vi "Periodic Tasks.vi"() -> ()   [LabVIEW 2012]
doc: "This VI runs in parallel to other tasks. It can contain as many user-defined periodic loops as you need. These can carry out PID or other sorts of timed response."
uses:
  <vilib>/Rock Robotics/WPI/Joystick/WPI_JoystickButtonState.ctl
  <vilib>/Rock Robotics/SystemInterfaces/Utilities/FPGA_UtilitiesLED Source.ctl
  <vilib>/Rock Robotics/SystemInterfaces/Utilities/FPGA_UtilitiesLED State.ctl
  <vilib>/Rock Robotics/WPI/Compressor/WPI_CompressorGetSetRefNum.vi
  Robot Global Data.vi
  <vilib>/Rock Robotics/WPI/RobotDrive/WPI_RobotDriveArcadeDrive_Standard(NoSaturation).vi
  <vilib>/Rock Robotics/WPI/Joystick/WPI_JoystickGetSetRefNum.vi
  <vilib>/Rock Robotics/WPI/RobotDrive/WPI_RobotDriveGetSetRefNum.vi
  <vilib>/Rock Robotics/WPI/Solenoid/WPI_SolenoidSetEnum.vi
  <vilib>/Rock Robotics/WPI/Solenoid/WPI_SolenoidValue.ctl
  <vilib>/Rock Robotics/Network Tables/SD Read Boolean.vi
panel:
  out "y":dbl
  out "x":dbl
  out "Axes":T1
  out "Climber operation":u64
  out "s2b":dbl
  out "s2a":dbl
  out "s1b":dbl
  out "s1a":dbl
  out "Buttons 2":T2
  out "Climber Arm Position":dbl
  out "Right Rate":dbl
  out "Left Rate":dbl
  out "Next Value":dbl
  out "Output 2":dbl
  out "Output":dbl
  out "axis 2 (y)":dbl
  out "Drive Ramp Constant Y":dbl
  out "Drive Mechanical Deadband Y":dbl
  out "Next X Value":dbl
  out "Prev X Value":dbl
  out "Next Y Value":dbl
  out "Prev Y Value":dbl
  out "Boolean":bool
  out "Buttons":T2
  out "front":bool
  out "rear":bool
  out "Button 3":bool
  in  "Climber Counter":u8
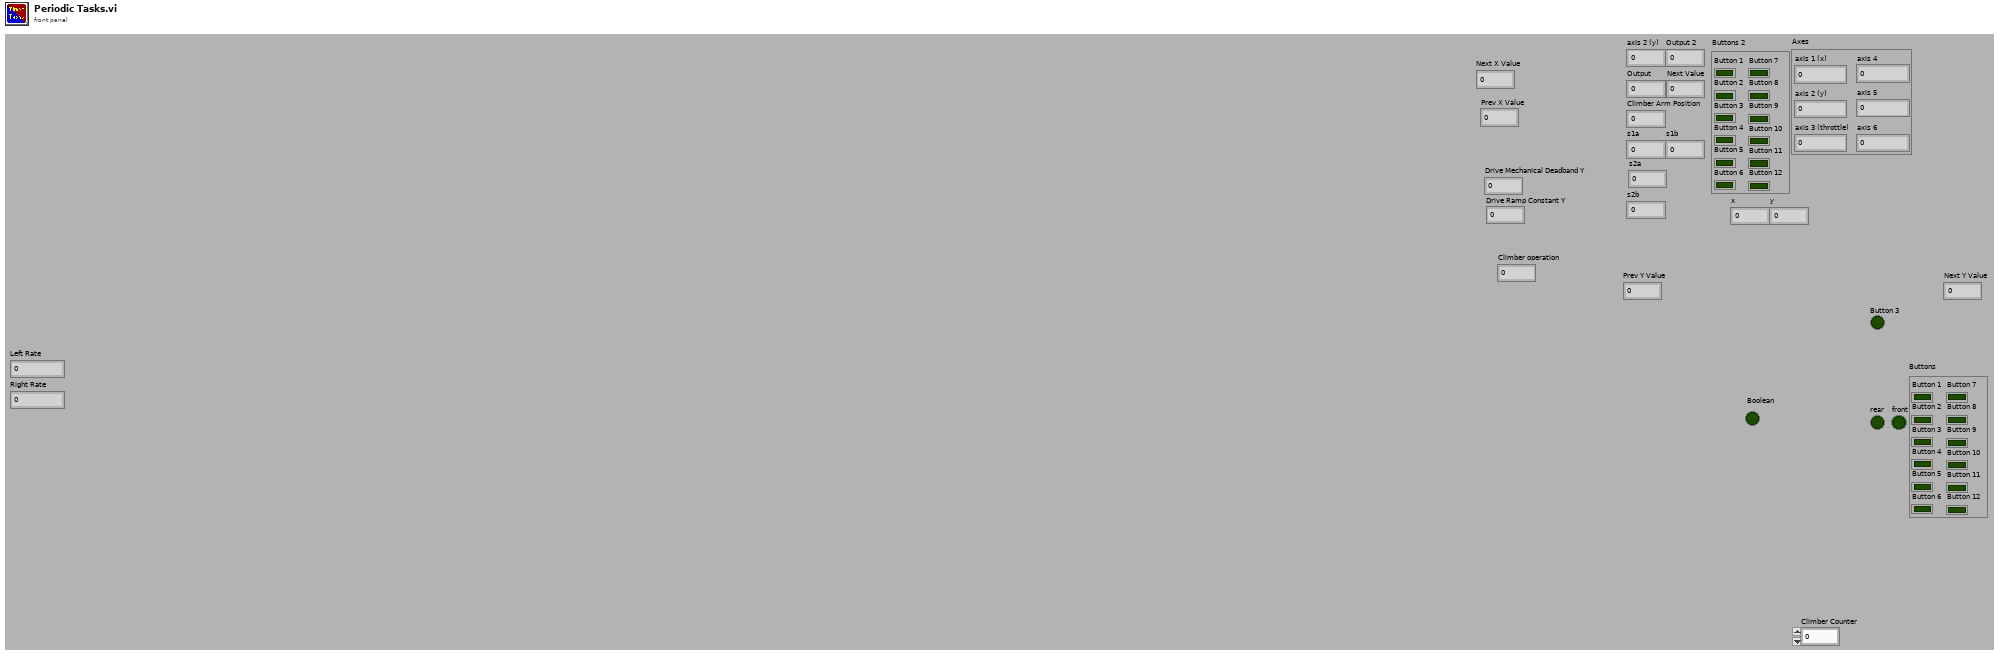
[diagram p1: front panel]
types:
  T1 = cluster{"axis 1 (x)":dbl, "axis 2 (y)":dbl, "axis 3 (throttle)":dbl, "axis 4":dbl, "axis 5":dbl, "axis 6":dbl}
  T2 = typedef "WPI_JoystickButtonState.ctl" = cluster{"Button 1":bool, "Button 2":bool, "Button 3":bool, "Button 4":bool, "Button 5":bool, "Button 6":bool, "Button 7":bool, "Button 8":bool, "Button 9":bool, "Button 10":bool, "Button 11":bool, "Button 12":bool}
  T3 = typedef "WPI_CompressorDevRef.ctl" = cluster{"DevStatus":errorcluster, "DigitalInputDevRef":T4, "RelayDevRef":T7}
  T4 = typedef "WPI_DigitalInputDevRef.ctl" = cluster{"DevStatus":errorcluster, "DIO Channel":T5, "Digital Module":T6}
  T5 = typedef "FPGA_DIOChannel.ctl" = enum8{"DIO 1", "DIO 2", "DIO 3", "DIO 4", "DIO 5", "DIO 6", "DIO 7", "DIO 8", "DIO 9", "DIO 10", "DIO 11", "DIO 12", "DIO 13", "DIO 14", "Invalid"}
  T6 = typedef "FPGA_TypedefDigitalModule.ctl" = enum16{"Digital Module 1", "Digital Module 2"}
  T7 = typedef "WPI_RelayDevRef.ctl" = cluster{"DevStatus":errorcluster, "Relay Channel":T8, "Digital Module":T6, "Relay Direction":T9}
  T8 = typedef "FPGA_DIORelayChannel.ctl" = enum8{"Relay 1", "Relay 2", "Relay 3", "Relay 4", "Relay 5", "Relay 6", "Relay 7", "Relay 8", "Invalid"}
  T9 = typedef "WPI_RelayDirection.ctl" = enum16{"Both directions", "Forward only", "Reverse only"}
  T10 = typedef "WPI_SolenoidValue.ctl" = enum16{"Off", "On", "Forward", "Reverse"}
  T11 = typedef "WPI_JoystickDevRef.ctl" = cluster{"Device":T12}
  T12 = typedef "WPI_JoystickDeviceEnum.ctl" = enum16{"USB 1", "USB 2", "USB 3", "USB 4", "Kinect 1", "Kinect 2"}
  T13 = typedef "WPI_SolenoidDevRef.ctl" = cluster{"DevStatus":errorcluster, "Solenoid Module":T14, "Forward Solenoid Channel":T15, "Reverse Solenoid Channel":T15}
  T14 = typedef "FPGA_TypedefSolenoidModule.ctl" = enum16{"Solenoid Module 1", "Solenoid Module 2"}
  T15 = typedef "WPI_SolenoidChannel.ctl" = enum8{"Solenoid 1", "Solenoid 2", "Solenoid 3", "Solenoid 4", "Solenoid 5", "Solenoid 6", "Solenoid 7", "Solenoid 8", "Invalid"}
  T16 = typedef "WPI_MotorControlDeviceRef.ctl" = cluster{"DeviceStatus":errorcluster, "Type":enum16{"PWM", "CAN"}, "PWM":cluster{"Digital Module":T6, "PWM Channel":T17, "DeadBand":T18}, "CAN":cluster{"Device Number":u8, "Control Mode":T19, "Semaphore":T20, "Max Vout":dbl}, "Invert":bool, "TransformRef":T21, "InvTransformRef":T21}
  T17 = typedef "FPGA_DIOPWMChannel.ctl" = enum8{"PWM 1", "PWM 2", "PWM 3", "PWM 4", "PWM 5", "PWM 6", "PWM 7", "PWM 8", "PWM 9", "PWM 10", "Invalid"}
  T18 = typedef "WPI_PWMDeadband.ctl" = cluster{"Name":string, "maxPositivePwm":i32, "minPositivePwm":i32, "centerPwm":i32, "maxNegativePwm":i32, "minNegativePwm":i32, "angularRange":u16}
  T19 = typedef "WPI_CANJaguar_ControlMode.ctl" = enum8{"Percent VBus", "Current", "Speed", "Position", "Voltage"}
  T20 = typedef "Semaphore RefNum" = refnum<k1>
  T21 = typedef "WPI_PWMTransform_ConPane.ctl" = refnum<vi>
  T22 = typedef "WPI_AnalogChannelDevRef.ctl" = cluster{"DevStatus":errorcluster, "Analog Module":T23, "Analog Channel":T24}
  T23 = typedef "FPGA_TypedefAnalogModule.ctl" = enum16{"Analog Module 1", "Analog Module 2"}
  T24 = typedef "FPGA_AIChannel.ctl" = enum8{"AI 1", "AI 2", "AI 3", "AI 4", "AI 5", "AI 6", "AI 7", "AI 8", "Invalid"}
  T25 = typedef "FPGA_UtilitiesLED State.ctl" = enum16{"Off", "On", "Toggle"}
  T26 = typedef "FPGA_UtilitiesLED Source.ctl" = enum16{"User LED", "FPGA LED"}
  T27 = typedef "WPI_EncoderDevRef.ctl" = cluster{"DevStatus":errorcluster, "EncoderIndex":T28, "CounterIndex":T29, "DistancePerCount":dbl, "Decoding Type":T30}
  T28 = typedef "FPGA_EncoderIdx.ctl" = enum8{"Enc 0", "Enc 1", "Enc 2", "Enc 3", "Invalid"}
  T29 = typedef "FPGA_CounterCtrSystemIndex.ctl" = enum8{"Ctr 0", "Ctr 1", "Ctr 2", "Ctr 3", "Ctr 4", "Ctr 5", "Ctr 6", "Ctr 7", "Invalid"}
  T30 = typedef "WPI_EncoderType.ctl" = enum16{"1x", "2x", "4x"}
  T31 = typedef "WPI_RobotDriveDevRef.ctl" = cluster{"DevStatus":errorcluster, "Motors[]":T16[], "Square Inputs":bool, "Max Output":dbl, "Isochronous":bool}
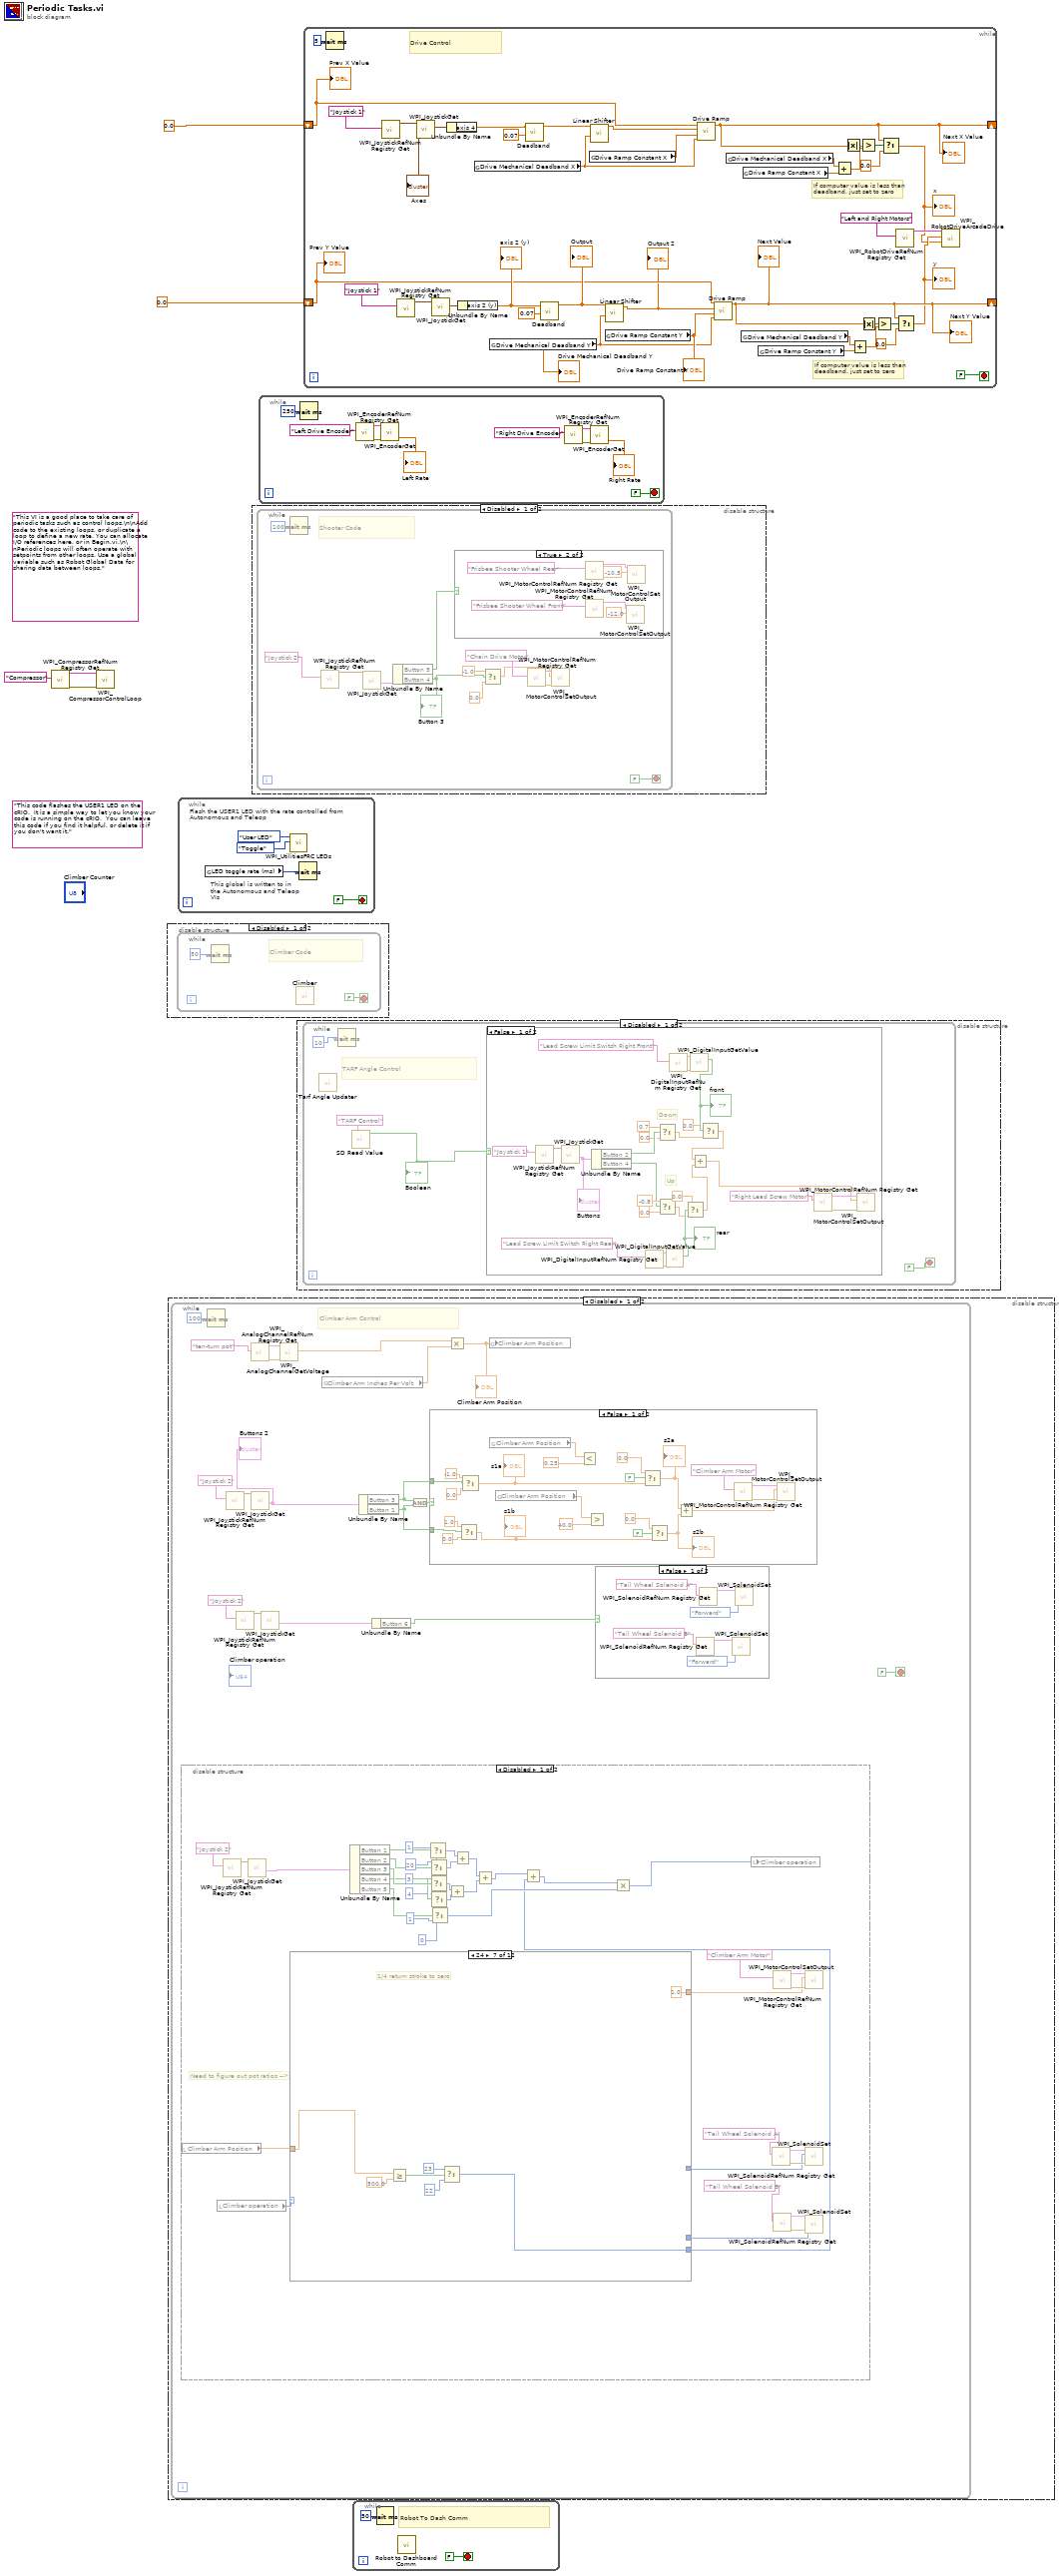
[diagram p0: block diagram]
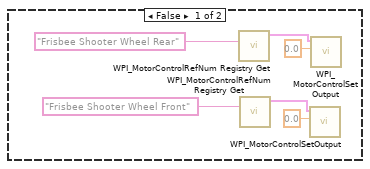
[diagram p2: hidden frame]
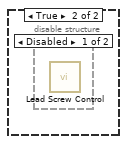
[diagram p4: hidden frame]
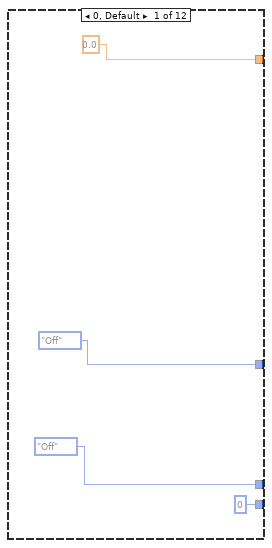
[diagram p7: hidden frame]
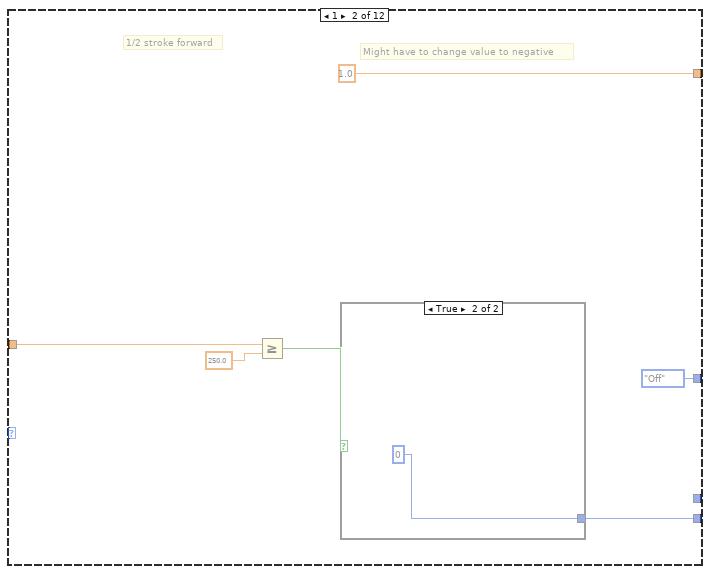
[diagram p8: hidden frame]
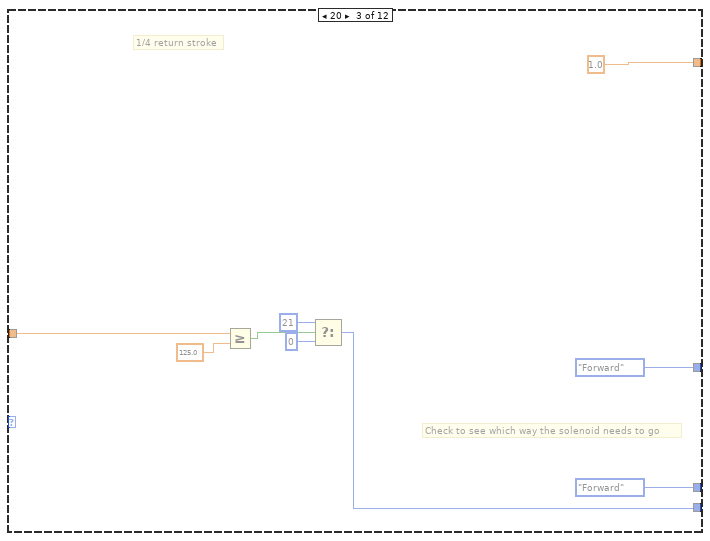
[diagram p10: hidden frame]
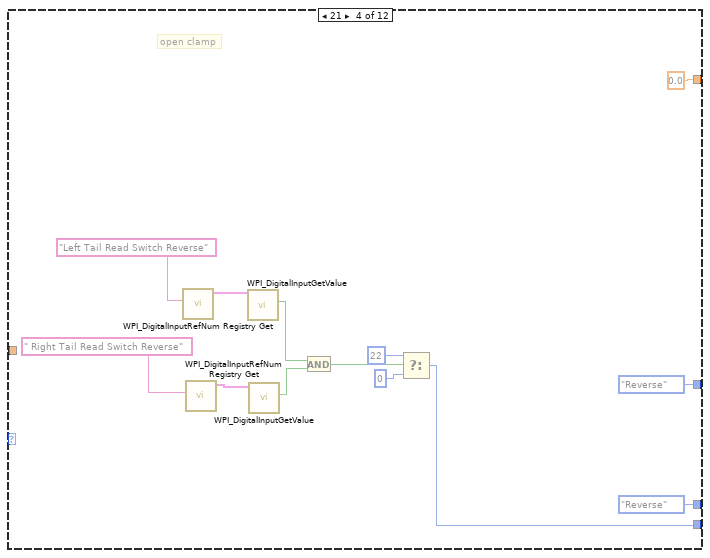
[diagram p11: hidden frame]
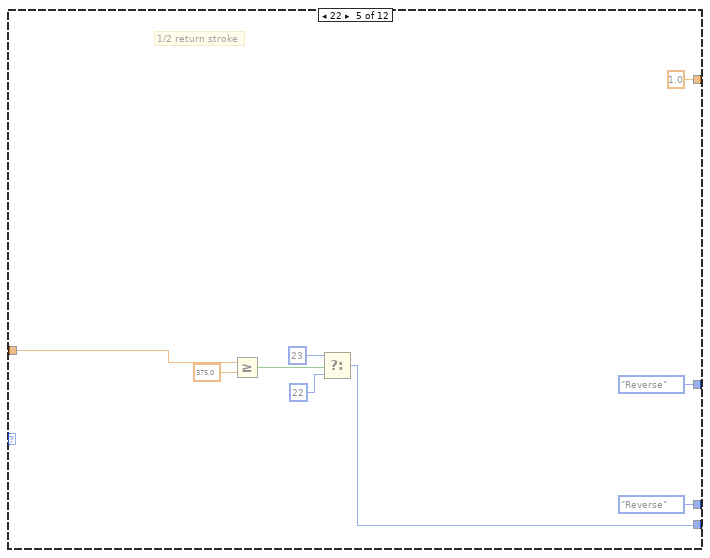
[diagram p12: hidden frame]
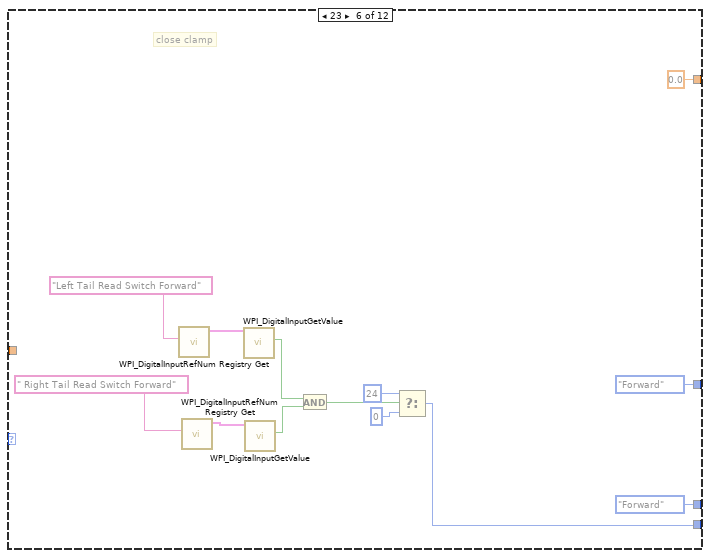
[diagram p13: hidden frame]
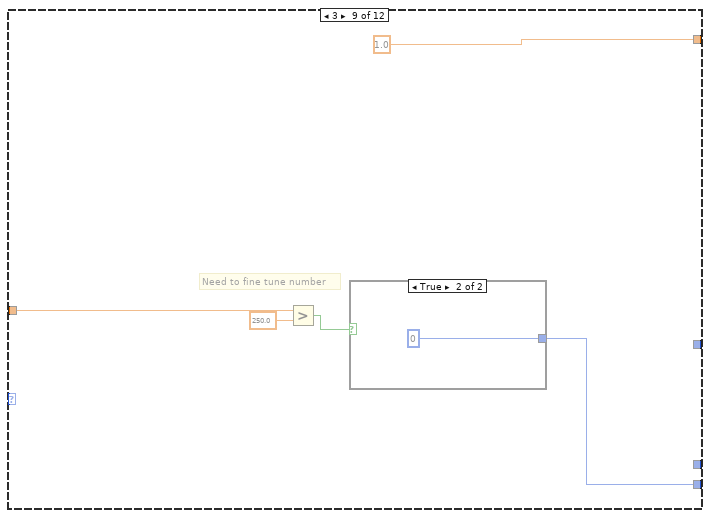
[diagram p15: hidden frame]
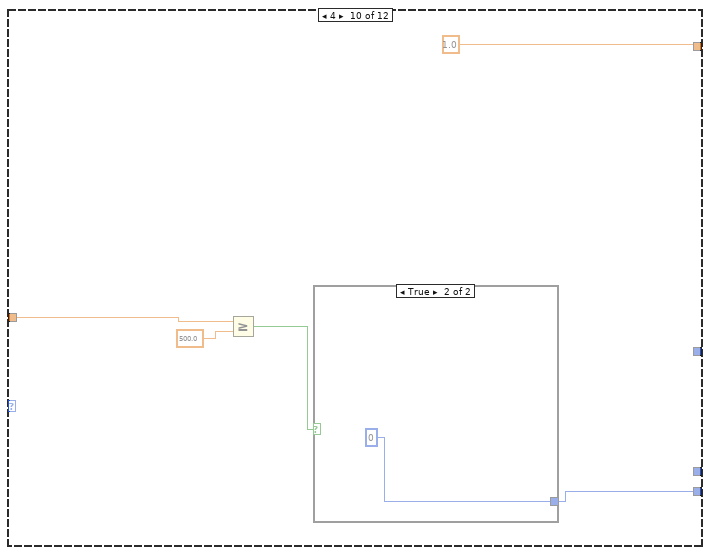
[diagram p17: hidden frame]
diagram:
  (unwired) "This code flashes the USER1 LED on the cRIO.  It is a simple way to let you know your code is running on the cRIO.  You can leave this code if you find it helpful, or delete it if you don't want it."
  (unwired) "This VI is a good place to take care of periodic tasks such as control loops.\n\nAdd code to the existing loops, or duplicate a loop to define a new rate. You can allocate I/O references here, or in Begin.vi.\n\nPeriodic loops will often operate with setpoints from other loops. Use a global variable such as Robot Global Data for sharing data between loops."
  n1 = call <vilib>:"WPI_CompressorRefNum Registry Get.vi"("refnum name"="Compressor") -> ("error out"=w4:errorcluster, "CompressorDevRef"=w3:T3)  [unwired: 9 in]
  n2 = call <vilib>:"WPI_CompressorControlLoop.vi"("error in (no error)"=w4, "CompressorDevRef"=w3) -> ()  [unwired: 10 in]
  n3 = disable-structure shown="Disabled" {
    frame Disabled {
      n4 = while {
        stop <- FALSE stop-if-true
        # "Climber Code"
        n5 = Wait (ms)(milliseconds to wait=u32 50) -> ()  [unwired: 1 out]
        n6 = call "Climber.vi"() -> ()  [unwired: 12 in]
      }
    }
    frame Enabled {
    }
  }
  n7 = disable-structure shown="Disabled" {
    frame Disabled {
      n8 = while {
        stop <- FALSE stop-if-true
        # "Climber Arm Control"
        n9 = disable-structure shown="Disabled" {
          frame Disabled {
            w44 = 0
            # "Need to figure out pot ratios -->"
            n10 = local read "Climber Arm Position"() -> (w29:dbl)
            n11 = local read "Climber operation"() -> (w42:u64)
            n12 = call <vilib>:"WPI_JoystickRefNum Registry Get.vi"("refnum name"="Joystick 2") -> ("JoystickDevRef"=w63:T11)  [unwired: 9 in, 1 out]
            n13 = call <vilib>:"WPI_JoystickGet.vi"("JoystickDevRef"=w63) -> ("Buttons"=w62:T2)  [unwired: 4 in, 2 out]
            n14 = case shown="24" w42 {
              tunnel: [WPI_SolenoidValue."Off" ("Value") WPI_SolenoidValue."Off" ("Value") WPI_SolenoidValue."Forward" ("Value") WPI_SolenoidValue."Reverse" ("Value") WPI_SolenoidValue."Reverse" ("Value") WPI_SolenoidValue."Forward" ("Value") _ _ _ _ _ _] -> w32
              tunnel: [WPI_SolenoidValue."Off" ("Value") _ WPI_SolenoidValue."Forward" ("Value") WPI_SolenoidValue."Reverse" ("Value") WPI_SolenoidValue."Reverse" ("Value") WPI_SolenoidValue."Forward" ("Value") _ _ _ _ _ _] -> w31
              tunnel: [0.0 ("Output") 1.0 ("Output") 1.0 ("Output") 0.0 ("Output") 1.0 ("Output") 0.0 ("Output") 1.0 ("Output") _ 1.0 ("Output") 1.0 ("Output") _ _] -> w30
              tunnel: w29 -> [_ w72 w83 _ w103 _ w122 _ w131 w135 _ _]
              tunnel: [u64 0 ("Climber operation") w70 w76 w85 w98 w108 w121 _ w128 w134 _ _] -> w27
              frame 0, Default {
              }
              frame 1 {
                # "1/2 stroke forward"
                # "Might have to change value to negative"
                n15 = Greater Or Equal?(x=w72, y=250.0) -> (x >= y?=w71:bool)
                n16 = case shown="True" w71 {
                  tunnel: [_ u64 0 ("Climber operation")] -> w70
                  frame False {
                  }
                  frame True {
                  }
                }
              }
              frame 20 {
                # "1/4 return stroke"
                # "Check to see which way the solenoid needs to go"
                n17 = Greater Or Equal?(x=w83, y=125.0) -> (x >= y?=w79:bool)
                n18 = Select(t=i64 21, s=w79, f=i64 0) -> (s? t:f=w76:i64)
              }
              frame 21 {
                # "open clamp"
                n19 = call <vilib>:"WPI_DigitalInputRefNum Registry Get.vi"("refnum name"="Left Tail Read Switch Reverse") -> ("DigitalInputDevRef"=w89:T4)  [unwired: 9 in, 1 out]
                n20 = call <vilib>:"WPI_DigitalInputRefNum Registry Get.vi"("refnum name"=" Right Tail Read Switch Reverse") -> ("DigitalInputDevRef"=w88:T4)  [unwired: 9 in, 1 out]
                n21 = call <vilib>:"WPI_DigitalInputGetValue.vi"("DigitalInputDevRef"=w89) -> ("Value"=w87:bool)  [unwired: 8 in, 2 out]
                n22 = call <vilib>:"WPI_DigitalInputGetValue.vi"("DigitalInputDevRef"=w88) -> ("Value"=w86:bool)  [unwired: 8 in, 2 out]
                n23 = And(x=w87, y=w86) -> (x .and. y?=w94:bool)
                n24 = Select(t=i64 22, s=w94, f=i64 0) -> (s? t:f=w85:i64)
              }
              frame 22 {
                # "1/2 return stroke"
                n25 = Greater Or Equal?(x=w103, y=375.0) -> (x >= y?=w101:bool)
                n26 = Select(t=i64 23, s=w101, f=i64 22) -> (s? t:f=w98:i64)
              }
              frame 23 {
                # "close clamp"
                n27 = call <vilib>:"WPI_DigitalInputRefNum Registry Get.vi"("refnum name"="Left Tail Read Switch Forward") -> ("DigitalInputDevRef"=w112:T4)  [unwired: 9 in, 1 out]
                n28 = call <vilib>:"WPI_DigitalInputRefNum Registry Get.vi"("refnum name"=" Right Tail Read Switch Forward") -> ("DigitalInputDevRef"=w111:T4)  [unwired: 9 in, 1 out]
                n29 = call <vilib>:"WPI_DigitalInputGetValue.vi"("DigitalInputDevRef"=w112) -> ("Value"=w110:bool)  [unwired: 8 in, 2 out]
                n30 = call <vilib>:"WPI_DigitalInputGetValue.vi"("DigitalInputDevRef"=w111) -> ("Value"=w109:bool)  [unwired: 8 in, 2 out]
                n31 = And(x=w110, y=w109) -> (x .and. y?=w117:bool)
                n32 = Select(t=i64 24, s=w117, f=i64 0) -> (s? t:f=w108:i64)
              }
              frame 24 {
                # "1/4 return stroke to zero"
                n33 = Greater Or Equal?(x=w122, y=500.0) -> (x >= y?=w125:bool)
                n34 = Select(t=i64 23, s=w125, f=i64 22) -> (s? t:f=w121:i64)
              }
              frame 25 {
                # "clearance forward"
              }
              frame 3 {
                # "Need to fine tune number"
                n35 = Greater?(x=w131, y=250.0) -> (0:w129:bool)
                n36 = case shown="True" w129 {
                  tunnel: [_ 0] -> w128
                  frame False {
                  }
                  frame True {
                  }
                }
              }
              frame 4 {
                n37 = Greater Or Equal?(x=w135, y=500.0) -> (x >= y?=w136:bool)
                n38 = case shown="True" w136 {
                  tunnel: [_ u64 0 ("Climber operation")] -> w134
                  frame False {
                  }
                  frame True {
                  }
                }
              }
              frame 5 {
              }
              frame 6 {
              }
            }
            n39 = Unbundle By Name(w62) -> ("Button 1"=w61:bool, "Button 2"=w60:bool, "Button 3"=w59:bool, "Button 4"=w58:bool, "Button 5"=w57:bool)
            n40 = Select(t=1, s=w61, f=w44) -> (s? t:f=w55:i32)
            n41 = Select(t=20, s=w60, f=w44) -> (s? t:f=w56:i32)
            n42 = Select(t=3, s=w59, f=w44) -> (s? t:f=w53:i32)
            n43 = Select(t=4, s=w58, f=w44) -> (s? t:f=w54:i32)
            n44 = Select(t=w44, s=w57, f=1) -> (s? t:f=w45:i32)
            n45 = Add(x=w53, y=w54) -> (x+y=w52:i32)
            n46 = Add(x=w55, y=w56) -> (x+y=w51:i32)
            n47 = Add(x=w51, y=w52) -> (x+y=w28:i32)
            n48 = Add(x=w28, y=w27) -> (x+y=w26:u64)
            n49 = Multiply(x=w26, y=w45) -> (x*y=w43:u64)
            n50 = local write "Climber operation"(w43) -> ()
            n51 = call <vilib>:"WPI_SolenoidRefNum Registry Get.vi"("refnum name"="Tail Wheel Solenoid A") -> ("error out"=w36:errorcluster, "SolenoidDevRef"=w35:T13)  [unwired: 9 in]
            n52 = call <vilib>:"WPI_MotorControlRefNum Registry Get.vi"("refnum name"="Climber Arm Motor") -> ("error out"=w38:errorcluster, "MotorControlDevRef"=w37:T16)  [unwired: 9 in]
            n53 = call <vilib>:"WPI_SolenoidRefNum Registry Get.vi"("refnum name"="Tail Wheel Solenoid B") -> ("error out"=w33:errorcluster, "SolenoidDevRef"=w34:T13)  [unwired: 9 in]
            n54 = call <vilib>:"WPI_MotorControlSetOutput.vi"("error in (no error)"=w38, "Output"=w30, "MotorControlDevRef"=w37) -> ()  [unwired: 6 in, 3 out]
            n55 = call-poly <vilib>:"WPI_SolenoidSet.vi"("error in (no error)"=w36, "Value"=w32, "SolenoidDevRef"=w35) -> ()  [unwired: 7 in, 2 out]
            n56 = call-poly <vilib>:"WPI_SolenoidSet.vi"("error in (no error)"=w33, "Value"=w31, "SolenoidDevRef"=w34) -> ()  [unwired: 7 in, 2 out]
          }
          frame Enabled {
          }
        }
        n57 = Wait (ms)(milliseconds to wait=u32 100) -> ()  [unwired: 1 out]
        n58 = call <vilib>:"WPI_JoystickRefNum Registry Get.vi"("refnum name"="Joystick 2") -> ("JoystickDevRef"=w13:T11)  [unwired: 9 in, 1 out]
        n59 = call <vilib>:"WPI_JoystickRefNum Registry Get.vi"("refnum name"="Joystick 2") -> ("JoystickDevRef"=w16:T11)  [unwired: 9 in, 1 out]
        n60 = call <vilib>:"WPI_AnalogChannelRefNum Registry Get.vi"("refnum name"="ten-turn pot") -> ("error out"=w22:errorcluster, "AIDeviceRef"=w21:T22)  [unwired: 9 in]
        n61 = call <vilib>:"WPI_JoystickGet.vi"("JoystickDevRef"=w13) -> ("Buttons"=w10:T2)  [unwired: 4 in, 2 out]
        "Buttons 2" <- w10
        n62 = call <vilib>:"WPI_JoystickGet.vi"("JoystickDevRef"=w16) -> ("Buttons"=w15:T2)  [unwired: 4 in, 2 out]
        n63 = call <vilib>:"WPI_AnalogChannelGetVoltage.vi"("error in (no error)"=w22, "AIDeviceRef"=w21) -> ("Voltage"=w20:dbl)  [unwired: 7 in, 2 out]
        n64 = global read "Robot Global Data.vi" "Climber Arm Inches Per Volt"() -> (w18:dbl)
        n65 = Unbundle By Name(w10) -> ("Button 3"=w9:bool, "Button 1"=w8:bool)
        n66 = Unbundle By Name(w15) -> ("Button 6"=w11:bool)
        n67 = And(x=w9, y=w8) -> (x .and. y?=w12:bool)
        n68 = case shown="False" w12 {
          tunnel: w9 -> [w156 _]
          tunnel: w8 -> [w151 _]
          frame False {
            n69 = Select(t=1.0, s=w151, f=0.0) -> (s? t:f=w141:dbl)
            "s1b" <- w141
            n70 = Select(t=-1.0, s=w156, f=0.0) -> (s? t:f=w142:dbl)
            "s1a" <- w142
            n71 = global read "Robot Global Data.vi" "Climber Arm Position"() -> (w149:dbl)
            n72 = global read "Robot Global Data.vi" "Climber Arm Position"() -> (w147:dbl)
            n73 = Less?(x=w149, y=0.25) -> ()  [unwired: 1 out]
            n74 = Greater?(x=w147, y=40.0) -> ()  [unwired: 1 out]
            n75 = Select(t=0.0, s=FALSE, f=w142) -> (s? t:f=w143:dbl)
            "s2a" <- w143
            n76 = Select(t=0.0, s=FALSE, f=w141) -> (s? t:f=w144:dbl)
            "s2b" <- w144
            n77 = Add(x=w143, y=w144) -> (x+y=w158:dbl)
            n78 = call <vilib>:"WPI_MotorControlRefNum Registry Get.vi"("refnum name"="Climber Arm Motor") -> ("error out"=w160:errorcluster, "MotorControlDevRef"=w159:T16)  [unwired: 9 in]
            n79 = call <vilib>:"WPI_MotorControlSetOutput.vi"("error in (no error)"=w160, "Output"=w158, "MotorControlDevRef"=w159) -> ()  [unwired: 6 in, 3 out]
          }
          frame True {
            n80 = call <vilib>:"WPI_MotorControlRefNum Registry Get.vi"("refnum name"="Climber Arm Motor") -> ("error out"=w164:errorcluster, "MotorControlDevRef"=w163:T16)  [unwired: 9 in]
            n81 = call <vilib>:"WPI_MotorControlSetOutput.vi"("error in (no error)"=w164, "Output"=0.0, "MotorControlDevRef"=w163) -> ()  [unwired: 6 in, 3 out]
          }
        }
        n82 = Multiply(x=w20, y=w18) -> (x*y=w19:dbl)
        "Climber Arm Position" <- w19
        n83 = global write "Robot Global Data.vi" "Climber Arm Position"(w19) -> ()
        n84 = case shown="False" w11 {
          frame False {
            n85 = call <vilib>:"WPI_SolenoidRefNum Registry Get.vi"("refnum name"="Tail Wheel Solenoid B") -> ("SolenoidDevRef"=w166:T13)  [unwired: 9 in, 1 out]
            n86 = call <vilib>:"WPI_SolenoidRefNum Registry Get.vi"("refnum name"="Tail Wheel Solenoid A") -> ("SolenoidDevRef"=w169:T13)  [unwired: 9 in, 1 out]
            n87 = call-poly <vilib>:"WPI_SolenoidSet.vi"("Value"=WPI_SolenoidValue."Forward", "SolenoidDevRef"=w166) -> ()  [unwired: 8 in, 2 out]
            n88 = call-poly <vilib>:"WPI_SolenoidSet.vi"("Value"=WPI_SolenoidValue."Forward", "SolenoidDevRef"=w169) -> ()  [unwired: 8 in, 2 out]
          }
          frame True {
            n89 = call <vilib>:"WPI_SolenoidRefNum Registry Get.vi"("refnum name"="Tail Wheel Solenoid B") -> ("SolenoidDevRef"=w172:T13)  [unwired: 9 in, 1 out]
            n90 = call <vilib>:"WPI_SolenoidRefNum Registry Get.vi"("refnum name"="Tail Wheel Solenoid A") -> ("SolenoidDevRef"=w175:T13)  [unwired: 9 in, 1 out]
            n91 = call-poly <vilib>:"WPI_SolenoidSet.vi"("Value"=WPI_SolenoidValue."Reverse", "SolenoidDevRef"=w172) -> ()  [unwired: 8 in, 2 out]
            n92 = call-poly <vilib>:"WPI_SolenoidSet.vi"("Value"=WPI_SolenoidValue."Reverse", "SolenoidDevRef"=w175) -> ()  [unwired: 8 in, 2 out]
          }
        }
      }
    }
    frame Enabled {
    }
  }
  n93 = while {
    stop <- FALSE stop-if-true
    # "This global is written to in the Autonomous and Teleop VIs"
    # "Flash the USER1 LED with the rate controlled from Autonomous and Teleop"
    n94 = global read "Robot Global Data.vi" "LED toggle rate (ms)"() -> (w177:u32)
    n95 = call <vilib>:"WPI_UtilitiesFRC LEDs.vi"("State"=FPGA_UtilitiesLED_State."Toggle", "LED Type"=FPGA_UtilitiesLED_Source."User LED") -> ()  [unwired: 1 in, 9 out]
    n96 = Wait (ms)(milliseconds to wait=w177) -> ()  [unwired: 1 out]
  }
  n97 = disable-structure shown="Disabled" {
    frame Disabled {
      n98 = while {
        stop <- FALSE stop-if-true
        # "Shooter Code"
        n99 = Wait (ms)(milliseconds to wait=u32 100) -> ()  [unwired: 1 out]
        n100 = call <vilib>:"WPI_JoystickRefNum Registry Get.vi"("refnum name"="Joystick 2") -> ("JoystickDevRef"=w190:T11)  [unwired: 9 in, 1 out]
        n101 = call <vilib>:"WPI_JoystickGet.vi"("JoystickDevRef"=w190) -> ("Buttons"=w189:T2)  [unwired: 4 in, 2 out]
        n102 = Unbundle By Name(w189) -> ("Button 5"=w181:bool, "Button 4"=w188:bool)
        "Button 3" <- w188
        n103 = case shown="True" w181 {
          frame False {
            n104 = call <vilib>:"WPI_MotorControlRefNum Registry Get.vi"("refnum name"="Frisbee Shooter Wheel Rear") -> ("MotorControlDevRef"=w197:T16)  [unwired: 9 in, 1 out]
            n105 = call <vilib>:"WPI_MotorControlRefNum Registry Get.vi"("refnum name"="Frisbee Shooter Wheel Front") -> ("MotorControlDevRef"=w196:T16)  [unwired: 9 in, 1 out]
            n106 = call <vilib>:"WPI_MotorControlSetOutput.vi"("Output"=0.0, "MotorControlDevRef"=w196) -> ()  [unwired: 7 in, 3 out]
            n107 = call <vilib>:"WPI_MotorControlSetOutput.vi"("Output"=0.0, "MotorControlDevRef"=w197) -> ()  [unwired: 7 in, 3 out]
          }
          frame True {
            n108 = call <vilib>:"WPI_MotorControlRefNum Registry Get.vi"("refnum name"="Frisbee Shooter Wheel Rear") -> ("MotorControlDevRef"=w203:T16)  [unwired: 9 in, 1 out]
            n109 = call <vilib>:"WPI_MotorControlRefNum Registry Get.vi"("refnum name"="Frisbee Shooter Wheel Front") -> ("MotorControlDevRef"=w202:T16)  [unwired: 9 in, 1 out]
            n110 = call <vilib>:"WPI_MotorControlSetOutput.vi"("Output"=-12.0, "MotorControlDevRef"=w202) -> ()  [unwired: 7 in, 3 out]
            n111 = call <vilib>:"WPI_MotorControlSetOutput.vi"("Output"=-10.5, "MotorControlDevRef"=w203) -> ()  [unwired: 7 in, 3 out]
          }
        }
        n112 = Select(t=-1.0, s=w188, f=0.0) -> (s? t:f=w182:dbl)
        n113 = call <vilib>:"WPI_MotorControlRefNum Registry Get.vi"("refnum name"="Chain Drive Motor") -> ("error out"=w184:errorcluster, "MotorControlDevRef"=w183:T16)  [unwired: 9 in]
        n114 = call <vilib>:"WPI_MotorControlSetOutput.vi"("error in (no error)"=w184, "Output"=w182, "MotorControlDevRef"=w183) -> ()  [unwired: 6 in, 3 out]
      }
    }
    frame Enabled {
    }
  }
  n115 = while {
    stop <- FALSE stop-if-true
    n116 = Wait (ms)(milliseconds to wait=u32 250) -> ()  [unwired: 1 out]
    n117 = call <vilib>:"WPI_EncoderRefNum Registry Get.vi"("refnum name"="Left Drive Encoder") -> ("error out"=w213:errorcluster, "EncoderDevRef"=w212:T27)  [unwired: 9 in]
    n118 = call <vilib>:"WPI_EncoderGet.vi"("error in (no error)"=w213, "EncoderDevRef"=w212) -> ("Rate"=→"Left Rate":dbl)  [unwired: 4 in, 5 out]
    n119 = call <vilib>:"WPI_EncoderRefNum Registry Get.vi"("refnum name"="Right Drive Encoder") -> ("error out"=w210:errorcluster, "EncoderDevRef"=w211:T27)  [unwired: 9 in]
    n120 = call <vilib>:"WPI_EncoderGet.vi"("error in (no error)"=w210, "EncoderDevRef"=w211) -> ("Rate"=→"Right Rate":dbl)  [unwired: 4 in, 5 out]
  }
  n121 = disable-structure shown="Disabled" {
    frame Disabled {
      n122 = while {
        stop <- FALSE stop-if-true
        # "TARF Angle Control"
        n123 = call "Tarf Angle Updater.vi"() -> ()  [unwired: 12 in]
        n124 = Wait (ms)(milliseconds to wait=u32 10) -> ()  [unwired: 1 out]
        n125 = call-poly <vilib>:"SD Read Value.vi"("Name"="TARF Control") -> ("Boolean"=w216:bool)  [unwired: 8 in, 2 out]
        "Boolean" <- w216
        n126 = case shown="False" w216 {
          frame False {
            # "Up"
            # "Down"
            n127 = call <vilib>:"WPI_JoystickRefNum Registry Get.vi"("refnum name"="Joystick 1") -> ("JoystickDevRef"=w245:T11)  [unwired: 9 in, 1 out]
            n128 = call <vilib>:"WPI_JoystickGet.vi"("JoystickDevRef"=w245) -> ("Buttons"=w244:T2)  [unwired: 4 in, 2 out]
            "Buttons" <- w244
            n129 = Unbundle By Name(w244) -> ("Button 2"=w239:bool, "Button 4"=w234:bool)
            n130 = call <vilib>:"WPI_DigitalInputRefNum Registry Get.vi"("refnum name"="Lead Screw Limit Switch Right Rear") -> ("error out"=w227:errorcluster, "DigitalInputDevRef"=w226:T4)  [unwired: 9 in]
            n131 = Select(t=0.7, s=w239, f=0.0) -> (s? t:f=w223:dbl)
            n132 = Select(t=-0.8, s=w234, f=0.0) -> (s? t:f=w221:dbl)
            n133 = call <vilib>:"WPI_DigitalInputGetValue.vi"("error in (no error)"=w227, "DigitalInputDevRef"=w226) -> ("Value"=w224:bool)  [unwired: 7 in, 2 out]
            "rear" <- w224
            n134 = call <vilib>:"WPI_DigitalInputRefNum Registry Get.vi"("refnum name"="Lead Screw Limit Switch Right Front") -> ("error out"=w231:errorcluster, "DigitalInputDevRef"=w230:T4)  [unwired: 9 in]
            n135 = Select(t=0.0 ("f"), s=w224, f=w221) -> (s? t:f=w233:dbl)
            n136 = call <vilib>:"WPI_DigitalInputGetValue.vi"("error in (no error)"=w231, "DigitalInputDevRef"=w230) -> ("Value"=w229:bool)  [unwired: 7 in, 2 out]
            "front" <- w229
            n137 = Select(t=0.0, s=w229, f=w223) -> (s? t:f=w232:dbl)
            n138 = Add(x=w232, y=w233) -> (x+y=w240:dbl)
            n139 = call <vilib>:"WPI_MotorControlRefNum Registry Get.vi"("refnum name"="Right Lead Screw Motor") -> ("error out"=w241:errorcluster, "MotorControlDevRef"=w242:T16)  [unwired: 9 in]
            n140 = call <vilib>:"WPI_MotorControlSetOutput.vi"("error in (no error)"=w241, "Output"=w240, "MotorControlDevRef"=w242) -> ()  [unwired: 6 in, 3 out]
          }
          frame True {
            n141 = disable-structure shown="Disabled" {
              frame Disabled {
                n142 = call "Lead Screw Control.vi"() -> ()  [unwired: 12 in]
              }
              frame Enabled {
              }
            }
          }
        }
      }
    }
    frame Enabled {
    }
  }
  n143 = while {
    shift-right: [w254] -> _
    shift-left: 0.0 ("Drive Mechanical Deadband") -> [w258]
    shift-right: [w249] -> _
    shift-left: 0.0 ("Drive Mechanical Deadband") -> [w253]
    stop <- FALSE stop-if-true
    # "If computer value is less than\ndeadband, just set to zero"
    # "If computer value is less than\ndeadband, just set to zero"
    # "Drive Control"
    n144 = Wait (ms)(milliseconds to wait=u32 5) -> ()  [unwired: 1 out]
    n145 = call <vilib>:"WPI_JoystickRefNum Registry Get.vi"("refnum name"="Joystick 1") -> ("JoystickDevRef"=w272:T11)  [unwired: 1 in, 9 out]
    n146 = call <vilib>:"WPI_JoystickRefNum Registry Get.vi"("refnum name"="Joystick 1") -> ("JoystickDevRef"=w285:T11)  [unwired: 1 in, 9 out]
    n147 = call <vilib>:"WPI_JoystickGet.vi"("JoystickDevRef"=w272) -> ("Axes"=w271:T1)  [unwired: 1 in, 5 out]
    "Axes" <- w271
    n148 = call <vilib>:"WPI_JoystickGet.vi"("JoystickDevRef"=w285) -> ("Axes"=w284:T1)  [unwired: 1 in, 5 out]
    n149 = Unbundle By Name(w271) -> ("axis 4"=w263:dbl)
    n150 = Unbundle By Name(w284) -> ("axis 2 (y)"=w261:dbl)
    "axis 2 (y)" <- w261
    n151 = global read "Robot Global Data.vi" "Drive Mechanical Deadband X"() -> (w255:dbl)
    n152 = global read "Robot Global Data.vi" "Drive Mechanical Deadband Y"() -> (w250:dbl)
    "Drive Mechanical Deadband Y" <- w250
    n153 = call "Deadband.vi"("Deadband"=0.07, "Input"=w263) -> ("Output"=w260:dbl)  [unwired: 9 in]
    n154 = call "Deadband.vi"("Deadband"=0.07, "Input"=w261) -> ("Output"=w259:dbl)  [unwired: 9 in]
    "Output" <- w259
    n155 = global read "Robot Global Data.vi" "Drive Ramp Constant X"() -> (w256:dbl)
    n156 = call "Linear Shifter.vi"("Shift"=w255, "Input"=w260) -> ("Output"=w257:dbl)  [unwired: 9 in]
    n157 = call "Linear Shifter.vi"("Shift"=w250, "Input"=w259) -> ("Output"=w252:dbl)  [unwired: 9 in]
    "Output 2" <- w252
    n158 = global read "Robot Global Data.vi" "Drive Ramp Constant Y"() -> (w251:dbl)
    "Drive Ramp Constant Y" <- w251
    n159 = call "Drive Ramp.vi"("Deadband"=w255, "Ramp Value"=w256, "Control Input"=w257, "Previous Value"=w258) -> ("Next Value"=w254:dbl)  [unwired: 7 in]
    "Next X Value" <- w254
    n160 = call "Drive Ramp.vi"("Deadband"=w250, "Ramp Value"=w251, "Control Input"=w252, "Previous Value"=w253) -> ("Next Value"=w249:dbl)  [unwired: 7 in]
    "Next Y Value" <- w249
    "Next Value" <- w249
    n161 = global read "Robot Global Data.vi" "Drive Mechanical Deadband X"() -> (w267:dbl)
    n162 = global read "Robot Global Data.vi" "Drive Mechanical Deadband Y"() -> (w276:dbl)
    n163 = global read "Robot Global Data.vi" "Drive Ramp Constant X"() -> (w266:dbl)
    n164 = global read "Robot Global Data.vi" "Drive Ramp Constant Y"() -> (w275:dbl)
    n165 = Add(x=w267, y=w266) -> (x+y=w265:dbl)
    n166 = Absolute Value(x=w254) -> (abs(x)=w270:dbl)
    n167 = Add(x=w276, y=w275) -> (x+y=w274:dbl)
    n168 = Greater?(x=w270, y=w265) -> (0:w269:bool)
    n169 = Absolute Value(x=w249) -> (abs(x)=w279:dbl)
    n170 = Greater?(x=w279, y=w274) -> (0:w278:bool)
    n171 = Select(t=w254, s=w269, f=0.0) -> (s? t:f=w247:dbl)
    "x" <- w247
    n172 = call <vilib>:"WPI_RobotDriveRefNum Registry Get.vi"("refnum name"="Left and Right Motors") -> ("RobotDriveDevRef"=w281:T31)  [unwired: 1 in, 9 out]
    n173 = Select(t=w249, s=w278, f=0.0) -> (s? t:f=w248:dbl)
    "y" <- w248
    n174 = call-poly <vilib>:"WPI_RobotDriveArcadeDrive.vi"("Y axis value"=w247, "X axis value"=w248, "RobotDriveDevRef"=w281) -> ()  [unwired: 6 in, 3 out]
    "Prev Y Value" <- w253
    "Prev X Value" <- w258
  }
  n175 = while {
    stop <- FALSE stop-if-true
    # "Robot To Dash Comm"
    n176 = Wait (ms)(milliseconds to wait=u32 50) -> ()  [unwired: 1 out]
    n177 = call "Robot to Dashboard Comm.vi"() -> ()  [unwired: 12 in]
  }
